vi "XL320_Configure Angle Limits.vi"(0 "VISA resource name":refnum<visa-resource-name>, 5 "Motor ID (0)":u8, 7 "Clockwise Angle Limit (0 deg)":dbl, 9 "Counter-Clockwise Angle Limit (300 deg)":dbl=300.0, 11 "error in (no error)":errorcluster) -> (4 "VISA resource name out":refnum<visa-resource-name>, 15 "error out":errorcluster)   [LabVIEW 2017, in "Dynamixel XL320.lvlib"]
doc: "Changes the ID of a motor."
uses:
  <instrlib>/Dynamixel XL320 (Drivers instrument)/Dynamixel XL320.lvlib
  <instrlib>/Dynamixel XL320 (Drivers instrument)/Public/Configure/XL320_Select_Action.ctl
panel:
  # "Ghislain REMY, IUT de Cachan, 2015 December 2015"
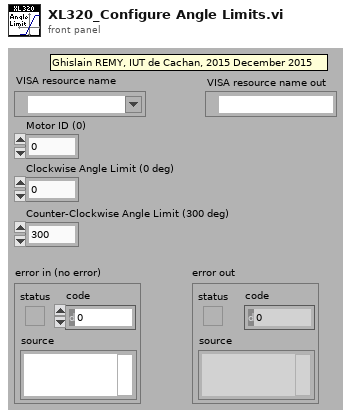
[diagram p1: front panel]
types:
  T1 = enum16{"big-endian, network order", "native, host order", "little-endian"}
  T2 = typedef "Dynamixel XL320.lvlib/XL320_Select_Action.ctl" = u8
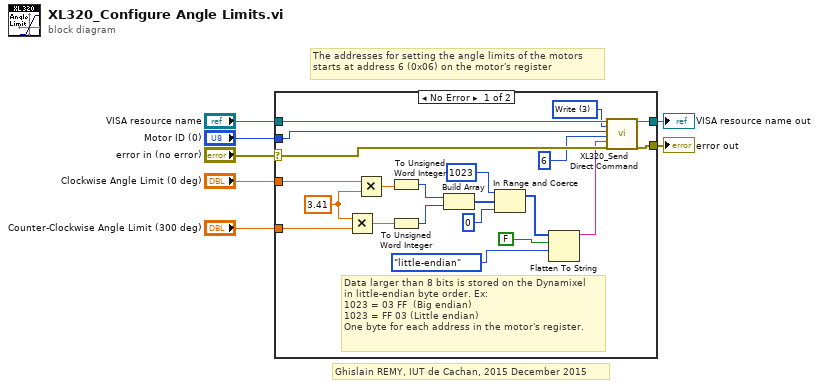
[diagram p0: block diagram]
diagram:
  # "Ghislain REMY, IUT de Cachan, 2015 December 2015"
  # "The addresses for setting the angle limits of the motors\nstarts at address 6 (0x06) on the motor's register"
  n1 = case shown="No Error" "error in (no error)" {
    selector: "error in (no error)" -> [w12 w30]
    tunnel: [w13 w30] -> w6
    tunnel: "VISA resource name" -> [w15 w29]
    tunnel: [w14 w29] -> w4
    tunnel: "Motor ID (0)" -> [w9 _]
    tunnel: "Clockwise Angle Limit (0 deg)" -> [w27 _]
    tunnel: "Counter-Clockwise Angle Limit (300 deg)" -> [w26 _]
    frame No Error {
      w8 = T2 3 items=["Ping"=1, "Read"=2, "Write"=3, "Registered Write"=4, "Action"=5, "Reset"=6, "Reboot"=8, "Status"=85, "Sync Read"=130, "Sync Write"=131, "Bulk Read"=146, "Bulk Write"=147] ("Select Action")
      w28 = 3.41
      # "Data larger than 8 bits is stored on the Dynamixel \nin little-endian byte order. Ex:\n1023 = 03 FF  (Big endian)\n1023 = FF 03 (Little endian)\nOne byte for each address in the motor's register."
      n2 = Multiply(x=w28, y=w26) -> (x*y=w22:dbl)
      n3 = Multiply(x=w27, y=w28) -> (x*y=w23:dbl)
      n4 = To Unsigned Word Integer(number=w23) -> (unsigned 16bit integer=w21:u16)
      n5 = To Unsigned Word Integer(number=w22) -> (unsigned 16bit integer=w20:u16)
      n6 = Build Array(w21, w20) -> (w19:u16[])
      n7 = In Range and Coerce(upper limit=u16 1023, x=w19, lower limit=u16 0) -> (coerced(x)=w18:u16[])  [unwired: 1 out]
      n8 = Flatten To String(anything=w18, prepend array or string size? (T)=FALSE, byte order (0:big-endian, network order)=T1."little-endian") -> (data string=w11:string)  [unwired: 1 in, 2 out]
      n9 = call <instrlib>:"XL320_Send Direct Command.vi"("VISA resource name"=w15, "Select Action"=w8, "Motor ID (0)"=w9, "Address"=u16 6, "Parameters"=w11, "Error in (no error)"=w12) -> ("VISA resource name out"=w14:refnum<visa-resource-name>, "Error out"=w13:errorcluster)  [unwired: 11 in, 1 out]
    }
    frame Error {
    }
  }
  "VISA resource name out" <- w4
  "error out" <- w6
